vi "fi.vi"(1 "q_input":dbl[](array[numeric]), 2 "constraints cluster":T1) -> (0 "fi":dbl[](array[numeric]))   [LabVIEW 2019]
panel:
  out "fi feasible":bool[](array[boolean])
  # "input : constraints cluster\n             q_input"
  # "output : fi, array, m*1"
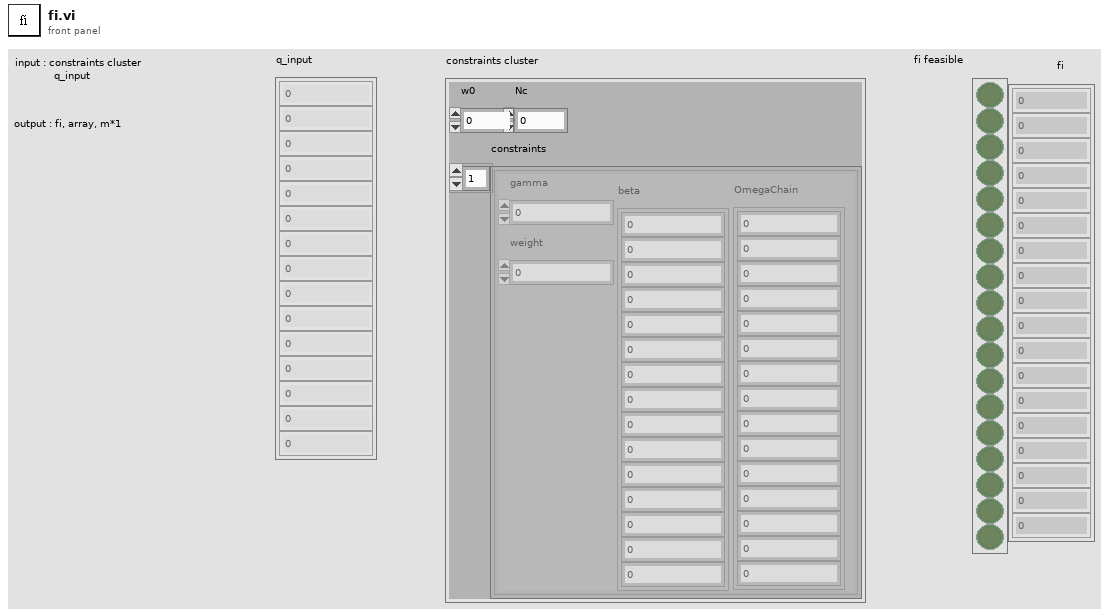
[diagram p1: front panel]
types:
  T1 = cluster{"w0":dbl, "constraints":cluster{"beta":dbl[], "gamma":dbl, "OmegaChain":dbl[], "weight":dbl}[], "Nc":i32}
  T2 = cluster{"beta":dbl[], "gamma":dbl, "OmegaChain":dbl[], "weight":dbl}[]
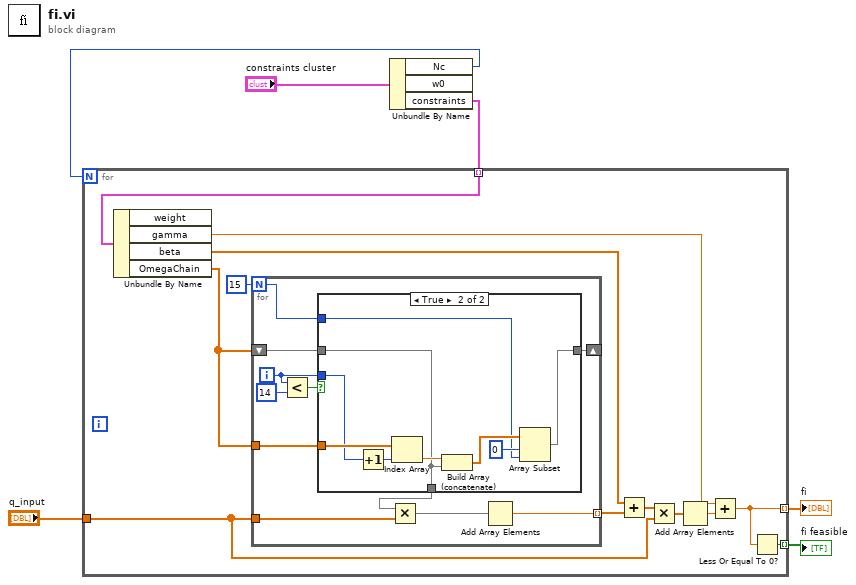
[diagram p0: block diagram]
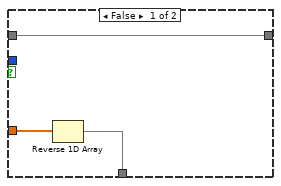
[diagram p2: hidden frame]
diagram:
  n1 = Unbundle By Name("constraints cluster") -> ("Nc"=w2:i32, "constraints"=w1:T2)  [unwired: 1 out]
  n2 = for {
    N: w2 -> [_]
    tunnel: "q_input" -> [w10]
    tunnel: [w14] -> w4 mode=indexing
    tunnel: [w16] -> w3 mode=indexing
    tunnel: w1 -> [w15] mode=indexing
    n3 = Unbundle By Name(w15) -> ("gamma"=w12:dbl, "beta"=w17:dbl[], "OmegaChain"=w13:dbl[])  [unwired: 1 out]
    n4 = for {
      N: 15 -> [w26]
      tunnel: w10 -> [w29]
      tunnel: [w27] -> w8 mode=indexing
      tunnel: w13 -> [w22]
      shift-right: [w19] -> _
      shift-left: w13 -> [w20]
      i -> [w23]
      n5 = Less?(x=w23, y=14) -> (x < y?=w24:bool)
      n6 = case shown="True" w24 {
        tunnel: w23 -> [_ w33]
        tunnel: w26 -> [_ w37]
        tunnel: w22 -> [w32 w36]
        tunnel: [w31 w35] -> w21
        tunnel: w20 -> [w30 w35]
        tunnel: [w30 w34] -> w19
        frame False {
          n7 = Reverse 1D Array(array=w32) -> (reversed array=w31:dbl[])
        }
        frame True {
          n8 = Increment(x=w33) -> (x+1=w38:i32)
          n9 = Index Array(array=w36, index=w38) -> (element=w39:dbl)
          n10 = Build Array (concatenate)(w39, w35) -> (w40:dbl[])
          n11 = Array Subset(array=w40, index=0, length=w37) -> (w34:dbl[])
        }
      }
      n12 = Multiply(x=w21, y=w29) -> (x*y=w28:dbl[])
      n13 = Add Array Elements(numeric array=w28) -> (sum=w27:dbl)
    }
    n14 = Add(x=w17, y=w8) -> (x+y=w9:dbl[])
    n15 = Multiply(x=w9, y=w10) -> (x*y=w7:dbl[])
    n16 = Add Array Elements(numeric array=w7) -> (sum=w11:dbl)
    n17 = Add(x=w12, y=w11) -> (x+y=w14:dbl)
    n18 = Less Or Equal To 0?(x=w14) -> (x <= 0?=w16:bool)
  }
  "fi" <- w4
  "fi feasible" <- w3
